vi "Actor Core.vi"(8 "error in":errorcluster, 11 "Nested in":refnum<class "UI ACTOR.lvclass">) -> (0 "error out":errorcluster, 3 "Actor out":refnum<class "Actor.lvclass">)   [LabVIEW 2020, in "UI ACTOR.lvlib" / "UI ACTOR.lvclass"]
doc: "(<B>Filename</B>: Actor Framework.lvlib:Actor.lvclass:Actor Core.vi)\n\nReceives messages to the actor, reacts to them, and initiates any error handling that may shut the actor down.\n\nDescendant classes may override this VI to append parallel tasks for the actor to complete while it handles messages. Overrides use the Call Parent Method node."
uses:
  UI ACTOR.lvclass
  C:/Program Files (x86)/National Instruments/LabVIEW 2020/vi.lib/ActorFramework/Actor/Actor.lvclass
  <vilib>/ActorFramework/Actor/Actor.lvclass
  <vilib>/ActorFramework/Actor/Actor.lvclass/Actor.ctl
  <vilib>/ActorFramework/Message Enqueuer/Message Enqueuer.lvclass/Message Enqueuer.ctl
  UI ACTOR.lvclass/UI ACTOR.ctl
  UI ACTOR Messages/Select Channel Msg/Select Channel Msg.lvclass/Select Channel Msg.ctl
  UI ACTOR Messages/Write and Read VISA Msg/Write and Read VISA Msg.lvclass/Write and Read VISA Msg.ctl
  <vilib>/ActorFramework/Message Enqueuer/Init from Existing Queue.vi
  <vilib>/ActorFramework/Message Enqueuer/Enqueue.vi
  <vilib>/ActorFramework/Stop Msg/Stop Msg.lvclass
  C:/Program Files (x86)/National Instruments/LabVIEW 2020/vi.lib/ActorFramework/Message/Message.lvclass
  UI ACTOR Messages/Read ADC UI Msg/Read ADC UI Msg.lvclass
  UI ACTOR Messages/Select Channel Msg/Select Channel Msg.lvclass
  UI ACTOR Messages/Write and Read VISA Msg/Write and Read VISA Msg.lvclass
  <vilib>/ActorFramework/Message Priority Queue/Priority Enqueue.vi
  <vilib>/Instr/_visa.llb/VISA Configure Serial Port (Instr).vi
  <vilib>/ActorFramework/Message Enqueuer/Message Enqueuer.lvclass
panel:
  in  "Channel":i32
  out "display":string
  out "String":string
  in  "OK Button":bool
  in  "VISA resource name":refnum<visa-resource-name>
  in  "WRITE PIN":bool
  in  "WRITE PORT":bool
  in  "READ  PIN":bool
  in  "READ PORT":bool
  in  "READ ADC":bool
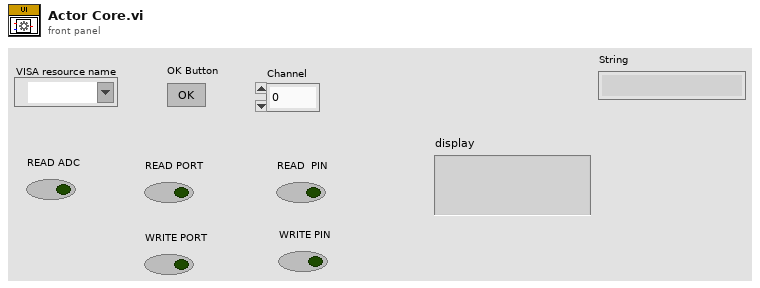
[diagram p1: front panel]
types:
  T1 = cluster{"Stop":refnum<user-event>, "String":refnum<user-event>, "display":refnum<user-event>}
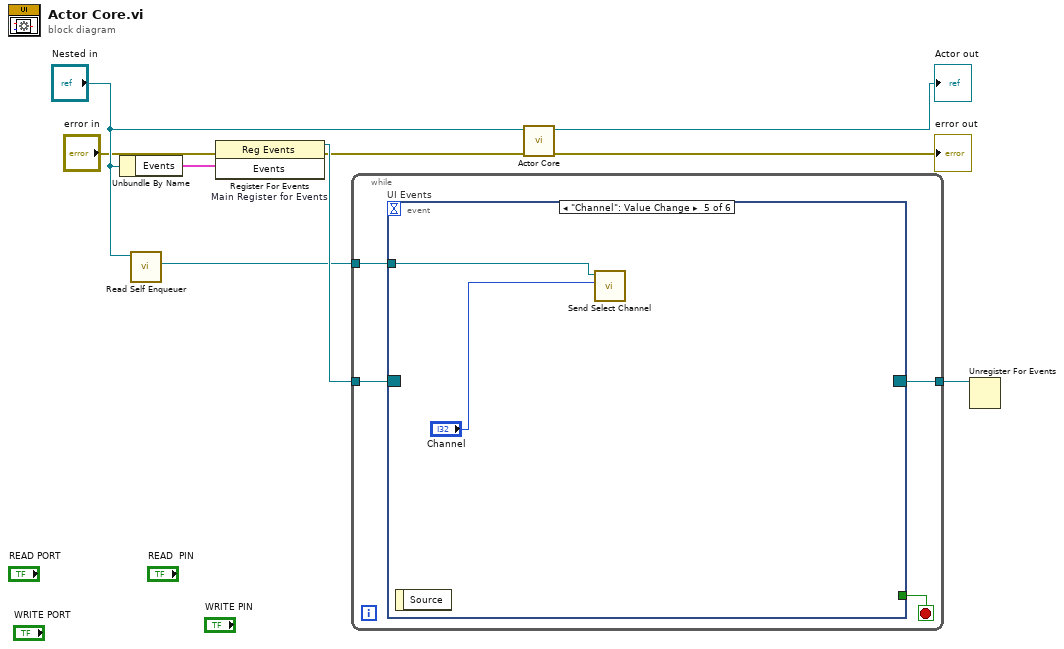
[diagram p0: block diagram]
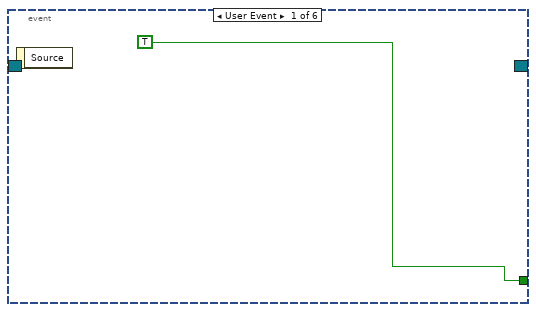
[diagram p2: hidden frame]
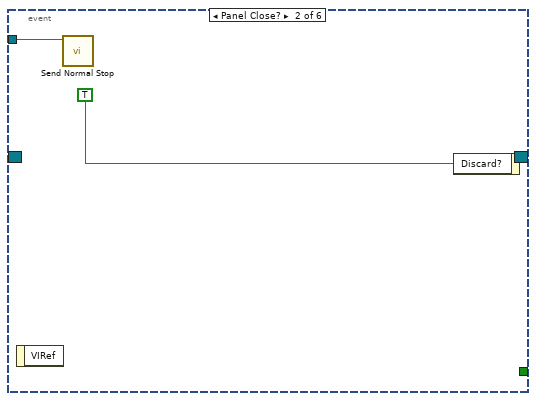
[diagram p3: hidden frame]
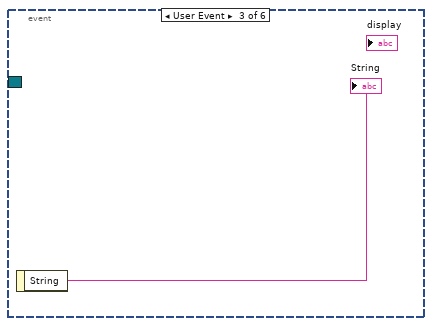
[diagram p4: hidden frame]
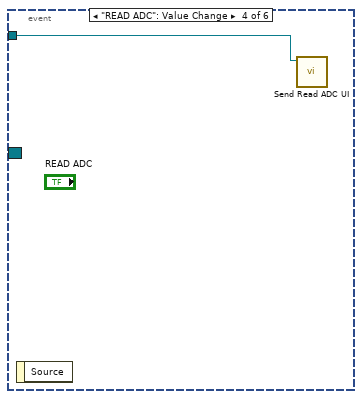
[diagram p5: hidden frame]
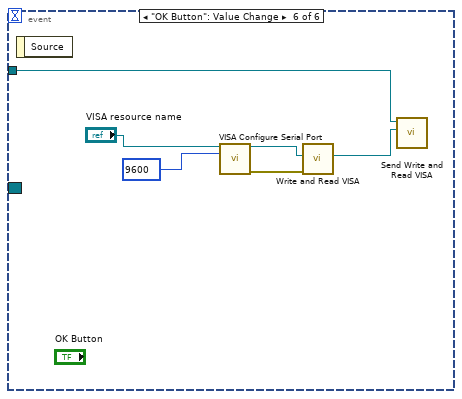
[diagram p6: hidden frame]
diagram:
  n1 = Unbundle By Name("Nested in") -> ("Events"=w6:T1)
  n2 = call <vilib>:"Read Self Enqueuer.vi"("Actor"="Nested in") -> ("Self Enqueuer"=w3:refnum<class "Message Enqueuer.lvclass">)  [unwired: 10 in]
  n3 = register-events "Main Register for Events"(error in="error in", w6) -> (reference out=w7:refnum<event-registration>, error out=w1:errorcluster)  [unwired: 1 in]
  n4 = while {
    tunnel: w7 -> [w13]
    tunnel: [w11] -> w5
    tunnel: w3 -> [w10]
    stop <- w12 stop-if-true
    n5 = event "UI Events" shown="[4] \"Channel\": Value Change" {
      selector: w13 -> [_ _ _ _ _ _]
      dyn-events: [_ _ _ _ _ _] -> w11
      timeout: _ -> [_ _ _ _ _ _]
      tunnel: [TRUE _ _ _ _ _] -> w12
      tunnel: w10 -> [_ w15 _ w18 w20 w22]
      event User Event {
        n6 = event-data() -> ()  [unwired: 1 in, 1 out]
      }
      event Panel Close? {
        n7 = event-data() -> ()  [unwired: 1 in, 1 out]
        n8 = call <vilib>:"Send Normal Stop.vi"("Message Enqueuer"=w15) -> ()  [unwired: 10 in, 1 out]
        n9 = event-data("Discard?"=TRUE) -> ()  [unwired: 1 in, 1 out]
      }
      event User Event {
        n10 = event-data() -> ("String"=→"String":string)  [unwired: 1 in]
      }
      event "READ ADC": Value Change {
        n11 = event-data() -> ()  [unwired: 1 in, 1 out]
        n12 = call "Send Read ADC UI.vi"("Message Enqueuer"=w18) -> ()  [unwired: 9 in, 2 out]
      }
      event "Channel": Value Change {
        n13 = event-data() -> ()  [unwired: 1 in, 1 out]
        n14 = call "Send Select Channel.vi"("Channel"="Channel", "Message Enqueuer"=w20) -> ()  [unwired: 8 in, 2 out]
      }
      event "OK Button": Value Change {
        n15 = event-data() -> ()  [unwired: 1 in, 1 out]
        n16 = call-poly "VISA Configure Serial Port"("VISA resource name"="VISA resource name", "baud rate (9600)"=u32 9600) -> ("VISA resource name out"=w24:refnum<visa-resource-name>, "error out"=w23:errorcluster)  [unwired: 12 in]
        n17 = call "Write and Read VISA.vi"("error in (no error)"=w23, "VISA resource name in"=w24) -> ("VISA resource name out"=w21:refnum<visa-resource-name>)  [unwired: 7 in, 2 out]
        n18 = call "Send Write and Read VISA.vi"("VISA resource name in"=w21, "Message Enqueuer"=w22) -> ()  [unwired: 8 in, 2 out]
      }
    }
  }
  n19 = call-parent "Actor Core.vi"("error in"=w1, "Actor in"="Nested in") -> ("error out"=→"error out":errorcluster, "Actor out"=→"Actor out":refnum<class "Actor.lvclass">)  [unwired: 8 in]
  n20 = Unregister For Events(event registration refnum=w5) -> ()  [unwired: 1 in, 1 out]
